vi "AlliGator Script Sequential ROIs Time-Gated Data Series Phasor Analysis.vi"(6 "AlliGator Data Series Type":T9, 8 "Error In":errorcluster, 9 "AlliGator Ctrl Refnums":T1, 10 "Path":path, 11 "Alligator Queue Elements in":T10[](array[typedef])) -> (0 "Error Out":errorcluster, 1 "Message":string, 2 "Time-Series Paths":path[](array[path]), 3 "Alligator Queue Elements out":T10[](array[typedef]))   [LabVIEW 2021, in "AlliGator Scripts.lvlib"]
doc: "Script performing phasor analysis of a different ROI for each dataset in a series. This is used for instance if the ROI list is representing the successive locations of an object being tracked across the dataset series."
uses:
  AlliGator Scripts.lvlib
  AlliGator Q Event.ctl
  AlliGator Action Engine.lvlib
  AlliGator Q Element.ctl
  Alligator Elements Order in Action Stack.ctl
  AlliGator Globals, Variables & Constants.lvlib
  AlliGator Variables List.ctl
  AlliGator Settings.lvlib
  AlliGator Settings List.ctl
  Graphs/XY Graph/XY Graph Plot Shift Method.ctl
  Graphs/XY Graph/XY Graph Add-Ons.lvlib
  Graphs/XY Graph/XY Graph Plot Shift Parameters.ctl
  Strings/Strings.lvlib
  Files/Files.lvlib
  AlliGator Phasor Ratio.lvlib
  AlliGator Files.lvlib
  AlliGator FLI Dataset Type.ctl
  AlliGator Add Action Array to Stack.vi
  Graphs/Plot Scales.ctl
  Graphs/LabVIEW Plot Interpolation.ctl
  Graphs/Graphs.lvlib
  Graphs/Plot Point Style.ctl
  Graphs/XY Graph/New Plot Information.ctl
  AlliGator Displayed Image.ctl
  AlliGator Source Image.lvlib
  Phasor/Phasor Standard Deviation Options.ctl
  Phasor/Phasor.lvlib
  Phasor/Phasor Ratio Type.ctl
  Variant/Variant to Data/Variant to Data.lvlib
  Variant/Variant to Data/Variant to Boolean.vi
  AlliGator Add Single Action to Stack.vi
  AlliGator ROIs.lvlib
  AlliGator ROI Manager Actions.ctl
  AlliGator ROI Selection Data.ctl
  <vilib>/Utility/miscctls.llb/LVPoint32TypeDef.ctl
  Graphs/XY Graph/XY Graph Refnum.ctl
  Graphs/XY Graph/XY Graph Mouse Click Event Data.ctl
  AlliGator Phasor Ratio at Mouse Location Data.ctl
  AlliGator Data Series Type.ctl
  AlliGator Dataset Ctrl Refnums.ctl
  AlliGator GUI.lvlib
  AlliGator Registered Events Ctrl Refnums.ctl
  Phasor/Phasor Calibration Type.ctl
  AlliGator Phasor Graph Ctrl Refnums.ctl
  AlliGator Phasor Plot Ctrl Refnums.ctl
  AlliGator State Indicator.ctl
  AlliGator Other Ctrl Refnums.ctl
  Histograms/Histogram Bin Position.ctl
  Histograms/Histogram Window.lvlib
  Histograms/Histogram Bin Option.ctl
  Histograms/Linear Histogram Options.ctl
  AlliGator Image Histogram Control Refnums.ctl
  AlliGator Decay Fit Map Control Refnums.ctl
  AlliGator Decay Fit Parameter Map.lvlib
  AlliGator Ctrl Refnums.ctl
  Fits/IRF(X)PSED/Decay Fit Parameters & Derived Quantities List.ctl
  Fits/Fits.lvlib
  AlliGator Main Window Tabs.ctl
panel:
  out "# Time Points":i32
  # "see the AlliGator License on the block diagram (Ctrl+E or Window:Show Block Diagram)"
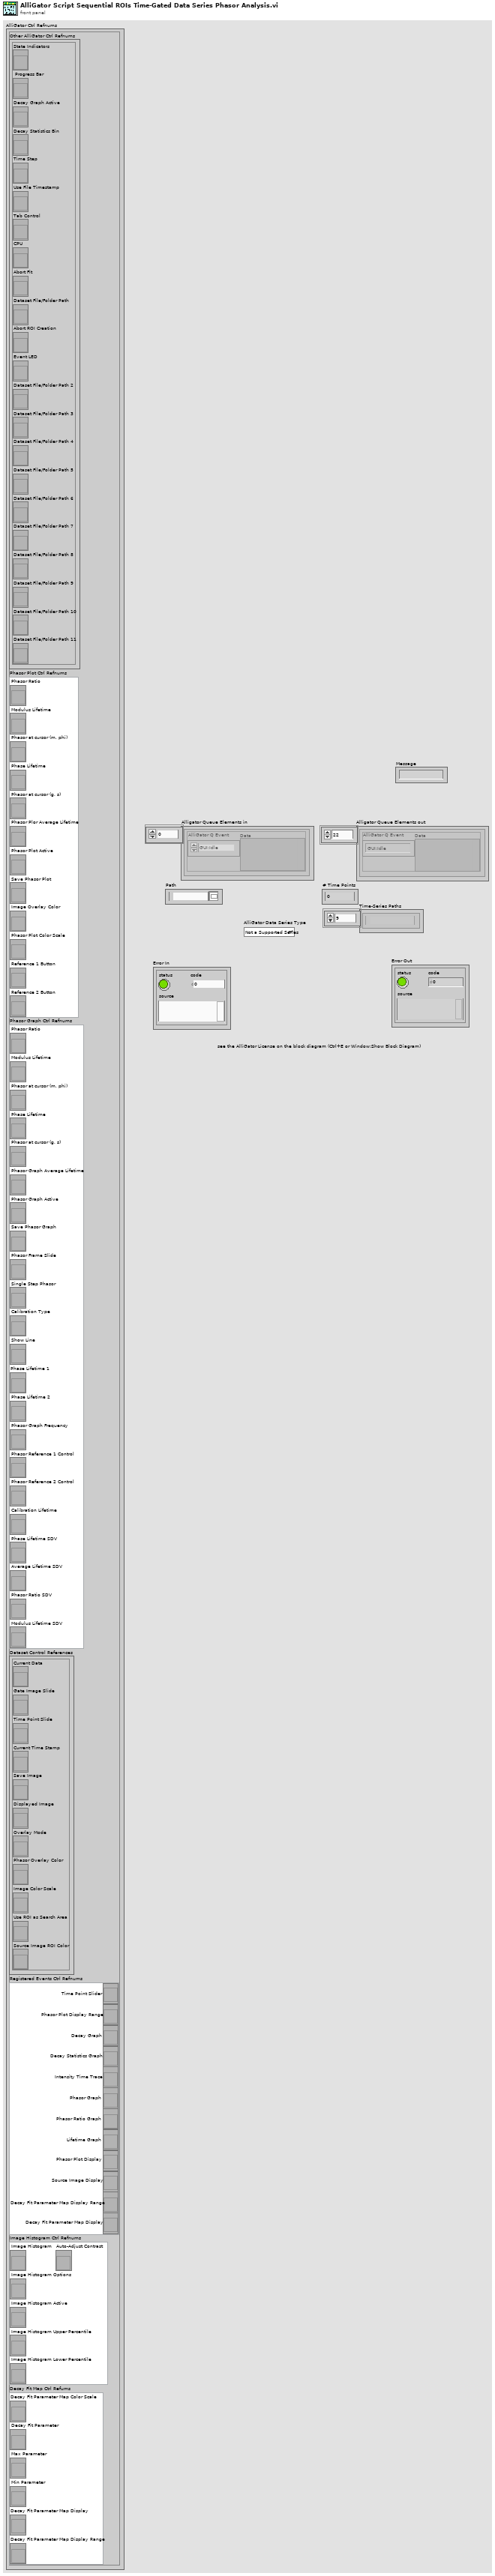
[diagram p1: front panel]
types:
  T1 = typedef "AlliGator GUI.lvlib/AlliGator Ctrl Refnums.ctl" = cluster{"Other AlliGator Ctrl Refnums":T2, "Phasor Plot Ctrl Refnums":T3, "Phasor Graph Ctrl Refnums":T4, "Dataset Control References":T5, "Registered Events Ctrl Refnums":T6, "Image Histogram Ctrl Refnums":T7, "Decay Fit Map Ctrl Refums":T8}
  T2 = typedef "AlliGator GUI.lvlib/AlliGator Other Ctrl Refnums.ctl" = cluster{"State Indicators":refnum<vi>, " Progress Bar":refnum<vi>, "Decay Graph Active":refnum<vi>, "Decay Statistics Bin":refnum<vi>, "Time Step":refnum<vi>, "Use File Timestamp":refnum<vi>, "Tab Control":refnum<vi>, "CPU":refnum<vi>, "Abort Fit":refnum<vi>, "Dataset File/Folder Path":refnum<vi>, "Abort ROI Creation":refnum<vi>, "Event LED":refnum<vi>, "Dataset File/Folder Path 2":refnum<vi>, "Dataset File/Folder Path 3":refnum<vi>, "Dataset File/Folder Path 4":refnum<vi>, "Dataset File/Folder Path 5":refnum<vi>, "Dataset File/Folder Path 6":refnum<vi>, "Dataset File/Folder Path 7":refnum<vi>, "Dataset File/Folder Path 8":refnum<vi>, "Dataset File/Folder Path 9":refnum<vi>, "Dataset File/Folder Path 10":refnum<vi>, "Dataset File/Folder Path 11":refnum<vi>}
  T3 = typedef "AlliGator GUI.lvlib/AlliGator Phasor Plot Ctrl Refnums.ctl" = cluster{"Phasor Ratio":refnum<vi>, "Modulus Lifetime":refnum<vi>, "Phasor at cursor (m, phi)":refnum<vi>, "Phase Lifetime":refnum<vi>, "Phasor at cursor (g, s)":refnum<vi>, "Phasor Plor Average Lifetime":refnum<vi>, "Phasor Plot Active":refnum<vi>, "Save Phasor Plot":refnum<vi>, "Image Overlay Color":refnum<vi>, "Phasor Plot Color Scale":refnum<vi>, "Reference 1 Button":refnum<vi>, "Reference 2 Button":refnum<vi>}
  T4 = typedef "AlliGator GUI.lvlib/AlliGator Phasor Graph Ctrl Refnums.ctl" = cluster{"Phasor Ratio":refnum<vi>, "Modulus Lifetime":refnum<vi>, "Phasor at cursor (m, phi)":refnum<vi>, "Phase Lifetime":refnum<vi>, "Phasor at cursor (g, s)":refnum<vi>, "Phasor Graph Average Lifetime":refnum<vi>, "Phasor Graph Active":refnum<vi>, "Save Phasor Graph":refnum<vi>, "Phasor Frame Slide":refnum<vi>, "Single Step Phasor":refnum<vi>, "Calibration Type":refnum<vi>, "Show Line":refnum<vi>, "Phase Lifetime 1":refnum<vi>, "Phase Lifetime 2":refnum<vi>, "Phasor Graph Frequency":refnum<vi>, "Phasor Reference 1 Control":refnum<vi>, "Phasor Reference 2 Control":refnum<vi>, "Calibration Lifetime":refnum<vi>, "Phase Lifetime SDV":refnum<vi>, "Average Lifetime SDV":refnum<vi>, "Phasor Ratio SDV":refnum<vi>, "Modulus Lifetime SDV":refnum<vi>}
  T5 = typedef "AlliGator GUI.lvlib/AlliGator Dataset Ctrl Refnums.ctl" = cluster{"Current Data":refnum<vi>, "Gate Image Slide":refnum<vi>, "Time Point Slide":refnum<vi>, "Current Time Stamp":refnum<vi>, "Save Image":refnum<vi>, "Displayed Image":refnum<vi>, "Overlay Mode":refnum<vi>, "Phasor Overlay Color":refnum<vi>, "Image Color Scale":refnum<vi>, "Use ROI as Search Area":refnum<vi>, "Source Image ROI Color":refnum<vi>}
  T6 = typedef "AlliGator GUI.lvlib/AlliGator Registered Events Ctrl Refnums.ctl" = cluster{"Time Point Slider":refnum<vi>, "Phasor Plot Display Range":refnum<vi>, "Decay Graph":refnum<vi>, "Decay Statistics Graph":refnum<vi>, "Intensity Time Trace":refnum<vi>, "Phasor Graph":refnum<vi>, "Phasor Ratio Graph":refnum<vi>, "Lifetime Graph":refnum<vi>, "Phasor Plot Display":refnum<vi>, "Source Image Display":refnum<vi>, "Decay Fit Parameter Map Display Range":refnum<vi>, "Decay Fit Parameter Map Display":refnum<vi>}
  T7 = typedef "AlliGator GUI.lvlib/AlliGator Image Histogram Control Refnums.ctl" = cluster{"Image Histogram":refnum<vi>, "Image Histogram Options":refnum<vi>, "Image Histogram Active":refnum<vi>, "Image Histogram Upper Percentile":refnum<vi>, "Image Histogram Lower Percentile":refnum<vi>, "Auto-Adjust Contrast":refnum<vi>}
  T8 = typedef "AlliGator Decay Fit Parameter Map.lvlib/AlliGator Decay Fit Map Control Refnums.ctl" = cluster{"Decay Fit Parameter Map Color Scale":refnum<vi>, "Decay Fit Parameter":refnum<vi>, "Max Parameter":refnum<vi>, "Min Parameter":refnum<vi>, "Decay Fit Parameter Map Display":refnum<vi>, "Decay Fit Parameter Map Display Range":refnum<vi>}
  T9 = typedef "AlliGator Files.lvlib/AlliGator Data Series Type.ctl" = enum16{"Not a Supported Series", "Gate Images Folder Series", "SwissSPAD 2 Dataset Series", "B&H FLI Dataset Series", "PicoQuant PTU FLI Dataset Series", "PicoQuant BIN FLI Dataset Series", "Piccolo hist BIN FLI Dataset Series", "HDF5 FLI Dataset Series"}
  T10 = typedef "AlliGator Action Engine.lvlib/AlliGator Q Element.ctl" = cluster{"AlliGator Q Event":T11, "Data":variant}
  T11 = typedef "AlliGator Action Engine.lvlib/AlliGator Q Event.ctl" = enum16{"---- Files ----", "Files:Set Batch Export Files To Save", "Files:Set Dataset Loading & Pre-processing Options", "Files:Check #Frames in Dataset", "Files:Increment Frame Index", "Files:Open Mask Image", "Files:Open White Light Image", "Files:Open Single Dataset", "Files:New Folder of Folders Selected", "Files:Load File (all Types)_Scriptable", "Files:Move Flattened Series to Folders Series", "Files:Select Folder", "Files:Load FLI Dataset", "Files:Load Swiss SPAD 1 Dataset", "Files:Load Swiss SPAD 2 Dataset", "Files:Load .sdt FLI Dataset", "Files:Load .ptu FLI Dataset", "Files:Load .bin FLI Dataset", "Files:Load Single Gate Image Folder", "Files:Load I/m/phi Dataset (deprecated)", "Files:Load Single Image", "Files:Subtract Background File", "Files:Export FLI Dataset", "Files:Load HDF5 FLI Dataset", "Files:Set Destination File Path", "Files:Save Mask Image", "Files:Batch Conversion", "Files:New Folder Selected", "Files:Close FLI Dataset", "Files:Close FLI Dataset Series", "Files:Close White Light Image", "Files:Close Mask Image", "---- FLI Dataset ----", "FLI Dataset:Channel Arithmetic", "FLI Dataset:Export Average Lifetime Map as ASCII", "FLI Dataset:Export User-Defined Quantity Map as ASCII", "FLI Dataset:Python Function FLI Dataset Event", "FLI Dataset:ROI Analysis", "FLI Dataset:Tilted Logistic Square Gated IRF Characteristics Map", "FLI Dataset:Logistic Square Gated IRF Characteristics Map", "FLI Dataset:Square Gated IRF Characteristics Map", "FLI Dataset:Multi-ROI Single-Pixel Phasor Analysis", "FLI Dataset:Multi-ROI Single-Pixel NLSF Analysis", "FLI Dataset:All ROIs IRF Extraction", "FLI Dataset:All ROIs Decay Fit Non-Interactive (Fast + Individual IRF)", "FLI Dataset:All ROIs Phasor Analysis", "FLI Dataset:All ROIs Decay Fit", "FLI Dataset:Fluorescence Decay Statistics", "FLI Dataset:Update Decay Statistics Graph", "FLI Dataset:Get Decay from ROI", "FLI Dataset:All ROIs Average Lifetimes", "---- FLI Dataset Series ----", "FLI Dataset Series:Sum All Datasets in Series", "FLI Dataset Series:Add Dataset to Accumulated Dataset", "FLI Dataset Series:Display Accumulated Dataset", "FLI Dataset Series:Clear Dataset Series Sum", "FLI Dataset Series:Time-Series Analysis (NLSF)", "FLI Dataset Series:Time-Series Analysis (Phasor)", "---- Image ----", "Image:Update Image Profile Plots", "Image:Image Histogram Cursor Move", "Image:Image Histogram", "Image:Image Contrast", "Image:Set Image Histogram Cursor Move Flag", "Image:Clear Image Overlay", "Image:Use ROI as Search Area", "Image:Set ROI Diameter", "Image:Save Image Data as TIFF", "Image:Save Displayed Image with Overlay", "Image:Save Image Overlay Only", "Image:Save Image as Hot Pixel Mask", "Image:Change Source Image Color Palette", "Image:Copy Image to Clipboard", "Image:Source Image ROI Selection", "Image:Delete All ROIs", "Image:Delete All Unselected ROIs", "Image:Delete ROI", "Image:Merge All ROIs", "Image:Store ROI", "Image:Source Image ROI Storage", "Image:Export ROI Description to Notebook", "Image:Save ROI", "Image:Load ROI", "Image:Paste ROI Definition", "Image:Clear ROI", "Image:Identify ROIs in Mask Image", "Image:Create Complementary ROI", "Image:Create Contour ROI", "Image:Create ROI(s) from Pixels with Peak above Min_Scriptable", "Image:Create ROI(s) from Pixels with Intensity above Min_Scriptable", "Image:Compute ROI Statistics", "Image:Delete ROI(s) based on ROI Characteristics", "Image:Create ROI Grid", "Image:ROI to Individual Pixel ROIs", "Image:Python Function Source Image Event", "Image:Show Phasor Calibration Map ROI Centers", "Image:Convert ROI to Mask Image", "Image:Mouse Move", "Image:Mouse Up", "Image:Set Source Image Mouse Move Flag", "Image:Add Scale Bar Overlay", "Image:Delete Existing ROIs Option", "---- Decay ----", "Decay:Clear IRF/Reference Plot", "Decay:Clear Local IRFs", "Decay:Add Decay to Graph", "Decay:Smoothen Plot", "Decay:Smoothen Plot Tail", "Decay:Average Selected Plots", "Decay:Extract IRF", "Decay:Optimal IRF Extraction", "Decay:Threshold IRF", "Decay:Fit to Model IRF", "Decay:Fit IRF to Square Gate", "Decay:Fit IRF to Logistic Square Gate", "Decay:Fit IRF to Tilted Logistic Square Gate", "Decay:Create Bounding Cursors Set", "Decay:Export Bounding Cursors Definition to Notebook", "Decay:Denoise Plot", "Decay:Compute Cumulative Function", "Decay:Use as Reference Decay", "Decay:Show Reference Decay/IRF", "Decay:Extrapolate Decay", "Decay:Create Head & Tail Bounding Cursors", "Decay:Store Cursor-defined Head & Tail Fractions", "Decay:Rebin Plot", "Decay:1-Normalize Decay", "Decay:[0-1]-Normalize Plot", "Decay:Straighten Decay", "Decay:Shift Decay", "Decay:Fold Decay", "Decay:Fit Decay", "Decay:Global Fit of Selected Decays", "Decay:Post Global Fit Script", "Decay:Add Global Fit Parameters to Graph", "Decay:Add Decay Parameter(s) to Plot (Graph)", "Decay:Export Decay to Phasor Graph", "Decay:Plot Decay Shifts", "Decay:Compute Average Lifetime", "Decay:Plot Convolution", "Decay:Graph Tip Strip Update", "---- Decay Statistics ----", "Decay Statistics:Tip Strip Update", "---- Intensity Time Trace ----", "Intensity Time Trace:Use File Timestamp", "Intensity Time Trace:Load Intensity Corrections File", "Intensity Time Trace:Clear Intensity Corrections File", "Intensity Time Trace:Tip Strip Update", "---- Phasor Plot ----", "Phasor Plot:Build Phasor Plot", "Phasor Plot:Change Phasor Plot Color Palette", "Phasor Plot:Adjust Phasor Plot Display Range", "Phasor Plot:Highlight Image ROI in Phasor Plot", "Phasor Plot:Save Phasor Plot Image with Overlay", "Phasor Plot:Export Complex Phasor Map", "Phasor Plot:Export Phasor Ratio Map", "Phasor Plot:Export Average Lifetime Map", "Phasor Plot:Compute Phase Lifetime Histogram", "Phasor Plot:Compute Phasor Ratio Histogram", "Phasor Plot:Compute Phase Lifetime vs Intensity Scatter Plot", "Phasor Plot:Weber 2-Component Decomposition", "Phasor Plot:Update Phasor Color Map Vertices", "Phasor Plot:Clear Phasor Overlay", "Phasor Plot:Use Segment Extremities as References", "Phasor Plot:Use UC/Segment Intersections as References", "Phasor Plot:Use UC/Principal Axis Intersections as References", "Phasor Plot:Use UC/Linear Fit Intersections as References", "Phasor Plot:Update Phasor Plot Reference", "Phasor Plot:Show Local Phasor Info in Phasor Plot", "Phasor Plot:Update Phasor Plot State", "Phasor Plot:Phasor Plot ROI Storage", "Phasor Plot:Phasor Plot ROI Selection", "Phasor Plot:Python Function Phasor Plot Event", "Phasor Plot:Overlay Phasor ROI, Ratio or Map in Source Image", "Phasor Plot:Compute Decay of Selected Phasors", "Phasor Plot:Phasor at Image Pixel", "Phasor Plot:Mouse Move", "Phasor Plot:Mouse Up", "Phasor Plot:Display Range Mouse Move", "Phasor Plot:Set Mouse Move Flag", "---- Phasor Graph ----", "Phasor Graph:Calibrated Phasor Map Series", "Phasor Graph:Whole Image Phasor Scatter Plot (Todo)", "Phasor Graph:Get Phasor Value", "Phasor Graph:Create New Phasor Plot Dialog", "Phasor Graph:Update Last Phasor Value", "Phasor Graph:Update Phasor (m, phi)", "Phasor Graph:Remove Single Phasor from Plot", "Phasor Graph:Add Single Phasor to Plot", "Phasor Graph:Remove Phasor Plot", "Phasor Graph:Remove Selected Phasor Plots", "Phasor Graph:Clear Phasor Data", "Phasor Graph:Clear Phasor Graph", "Phasor Graph:Cursor Move", "Phasor Graph:Draw Cursor Connecting Line", "Phasor Graph:Clear Cursor Connecting Line", "Phasor Graph:Find UC Intersection", "Phasor Graph:Use UC/Cursor-Defined Line Intersections", "Phasor Graph:Use Selected Plots Fitted Line/UC Intersections", "Phasor Graph:Use Selected Plots Principal Axis/UC Intersections", "Phasor Graph:Show Single Phasor", "Phasor Graph:Save Single Phasor Plot", "Phasor Graph:Save All Phasor Plots", "Phasor Graph:Load Phasor Plot(s)", "Phasor Graph:Phasor Multiplication", "Phasor Graph:Compute Average Phasor", "Phasor Graph:Compute Multiple Average Phasors (Selected Plots)", "Phasor Graph:Export Single Phasor Plot Phase Lifetimes", "Phasor Graph:Phase Lifetime Trajectory", "Phasor Graph:Phase Lifetime vs Intensity Scatter Plot (deprecated)", "Phasor Graph:Parameter 2 vs Parameter 1 Scatter Plot", "Phasor Graph:Use Cursor n Location", "Phasor Graph:Set Reference n to Current Phase Lifetime Value", "Phasor Graph:Set Reference n to Lifetime Value", "Phasor Graph:Set Cursor n Location", "Phasor Graph:Save Phasor Graph Image", "Phasor Graph:Update SEPL Plot", "Phasor Graph:Export Single Phasor Plot Data", "Phasor Graph:Export Selected Phasor Plots Data", "Phasor Graph:Python Function Phasor Graph Event", "Phasor Graph:Tip Strip Update", "---- Calibration ----", "Calibration:Set Calibration Type", "Calibration:Load/Save Phasor Calibration", "Calibration:Load/Save Phasor Calibration Series", "Calibration:Load/Save Phasor Calibration Map", "Calibration:Use as Calibration", "Calibration:Compute Optimal Calibration from Phasor References", "Calibration:Clear Phasor Calibration", "Calibration:Single Phasor Calibration Information", "Calibration:Use as Calibration Series", "Calibration:Use as Calibration Map", "Calibration:Clear Calibration Series", "Calibration:Phasor Calibration Series Information", "Calibration:Clear Calibration Map", "Calibration:Phasor Calibration Map Information", "Calibration:Apply Phasor Calibration", "Calibration:Update Single Plot Calibration", "Calibration:Update Multiple Plots Calibration", "Calibration:Clear Single Plot Calibration", "Calibration:Clear All Plots Calibrations", "Calibration:Clear Plot(s) Calibration(s)?", "Calibration:Phasor Calibration Maps (# Gates Series)", "---- Phasor Ratio ----", "Phasor Ratio:Clear Reference n", "Phasor Ratio:Toggle Selected Plot(s)  Lock to Reference 1", "Phasor Ratio:Use as Reference n", "Phasor Ratio:Send Reference n to Notebook", "Phasor Ratio:Toggle Selected Plot(s)  Lock to Reference 2", "Phasor Ratio:Compute Phasor Ratio at Mouse Location", "Phasor Ratio:Compute Phasor Plot's Average Phasor Ratio", "Phasor Ratio:Compute Time-Series Phasor Ratios", "Phasor Ratio:Fit Line to Phasor Ratio Plot", "Phasor Ratio:Save References", "Phasor Ratio:Load References", "Phasor Ratio:Update Phasor Reference 1", "Phasor Ratio:Update Phasor Reference 2", "Phasor Ratio:Move Cursor n to Reference n", "Phasor Ratio:Use as Phasor Reference 1 Lifetime", "Phasor Ratio:Use as Phasor Reference 2 Lifetime", "Phasor Ratio:Export Phasor Ratio Map as ASCII", "Phasor Ratio:Tip Strip Update", "---- Lifetime & Other Parameters Graph ----", "Lifetime:Tip Strip Update", "---- Decay Fit Parameter Map ----", "Decay Fit Parameter Map:Export ROI NLSF Data as ASCII", "Decay Fit Parameter Map:Set Decay Fit  Parameter Map Selection", "Decay Fit Parameter Map:Build Decay Fit Parameter Map", "Decay Fit Parameter Map:Change Decay Fit Parameter Map Color Palette", "Decay Fit Parameter Map:Export Decay Fit Parameter Map Data as ASCII", "Decay Fit Parameter Map:Export All Decay Fit Parameter Maps Data as ASCII", "Decay Fit Parameter Map:Send Map Data to Lifetime Graph", "Decay Fit Parameter Map:Save Decay Fit Parameter Map Image", "Decay Fit Parameter Map:Save-Load IRFs & Fit Data", "Decay Fit Parameter Map:Update Local Decay Plots", "Decay Fit Parameter Map:Python Function Decay Fit Parameters Map Event", "Decay Fit Parameter Map:Overlay Decay Fit Parameter Map in Source Image", "Decay Fit Parameter Map:Plot Map Data vs Intensity", "Decay Fit Parameter Map:Mouse Up", "Decay Fit Parameter Map:Display Range Mouse Move", "---- Generic Graph ----", "Generic Graph:Generic XY Graph Event", "Generic Graph:Python Function XY Graph Event", "Generic Graph:New Plot", "Generic Graph:Save Plot", "Generic Graph:XY Plot Histogram", "Generic Graph:Set XY Graph Plot Name", "Generic Graph:Set Last Cursor Style", "Generic Graph:Tip Strip Update", "---- GUI ----", "GUI:Start Script", "GUI:Type of Displayed Image Changed", "GUI:Gate Image Slide Changed", "GUI:Show Busy Icon", "GUI:Show Busy Icon & Abort Button", "GUI:Hide Busy Icon", "GUI:Hide Busy Icon & Abort Button", "GUI:Abort", "GUI:End Script", "GUI:Start Timing", "GUI:End Timing", "GUI:Set State Indicator", "GUI:Send Parameters JSON Strings to Clipboard", "GUI:Set Gate Step", "GUI:Idle", "GUI:Initialization", "GUI:Quit", "GUI:Increment Dataset Index", "GUI:Set Dataset Index to -1", "GUI:Time Series Slider Moved", "GUI:Time Series Slider Changed", "GUI:Toggle Playback or Loop", "GUI:Playback Script", "GUI:Set Phasor Frequency", "GUI:Open Window", "GUI:Start Test Script", "GUI:End Test Script", "DEBUG"}
  T12 = typedef "Phasor.lvlib/Phasor Ratio Type.ctl" = enum32{"Intensity-weighted", "Amplitude-weighted"}
  T13 = typedef "AlliGator Settings.lvlib/AlliGator Settings List.ctl" = enum16{"GUI:Visible Settings Tab", "GUI:Last Run Version", "Source Image:Use Image Histogram for Contrast", "Source Image:Low Count Pixels Rejection Options", "Source Image:High Count Pixels Rejection Options", "Source Image:Use Image Brightness", "Source Image:Blend Overlay with Image Background", "Source Image:Use Fixed ROI Diameter", "Source Image:ROI Diameter", "Source Image:ROI Center Color", "Source Image:Peak Threshold", "Source Image:Intensity Threshold", "Source Image:Image Binning Options", "Source Image:Image Smoothing Options", "Source Image:Image Histogram Active", "Source Image:Invert Binary Mask", "Source Image:Hot Pixel Removal", "Source Image:Overlay Analyzed ROI Center", "Source Image:Auto-Adjust Contrast", "Source Image:Histogram Lower Percentile", "Source Image:Histogram Upper Percentile", "Source Image:Save Source Image", "Source Image:Scale Bar Options", "Source Image:Image Resolution (Pixel Size)", "Source Image:Flatfield Correction", "Source Image:Show Dead Left Columns Correction", "Source Image:Dead Left Columns Correction", "Source Image:Image Pre-Processing Operations Order", "Data Information:Gate Width", "Data Information:Nanotime Gate Separation", "Data Information:Macrotime Gate Separation", "Data Information:Gate Step", "Data Information:# Gates", "Data Information:Gate Image Exposure", "Data Information:Gate Image Integration", "Data Information:Gates to Skip", "Data Information:Gates to Keep", "Data Information:Define Gates to", "Data Information:Channel Name", "Data Information:Available Channel Names", "Data Information:Channel Arithmetic", "Data Information:Background File Subtraction", "Data Information:Background File", "Data Information:Background Scaling Factor", "Data Information:Background Pile-up Correction", "Data Information:Background Pixel Well Capacity", "Data Information:Laser Period", "Data Information:SYNC Period", "Data Information:Pile-up Correction", "Data Information:Pixel Well Capacity", "Data Information:Dataset Scaling Factor", "Fluorescence Decay_Decay Pre-Processing:Reverse Gates", "Fluorescence Decay_Decay Pre-Processing:Verbose Decay Pre-Processing", "Fluorescence Decay_Decay Pre-Processing:Use Decay Pre-Processing", "Fluorescence Decay_Decay Pre-Processing:Background Subtraction", "Fluorescence Decay_Decay Pre-Processing:Background Definition Range", "Fluorescence Decay_Decay Pre-Processing:Baseline Subtraction Method", "Fluorescence Decay_Decay Pre-Processing:Decay Pre-Processing Operations Order", "Fluorescence Decay_Decay Pre-Processing:Smoothing Parameter", "Fluorescence Decay_Decay Pre-Processing:Shift Decay", "Fluorescence Decay_Decay Pre-Processing:Decay Shift Parameters", "Fluorescence Decay_Decay Pre-Processing:Fold Decay", "Fluorescence Decay_Decay Pre-Processing:# Folds", "Fluorescence Decay_Decay Pre-Processing:1-Normalize Decay", "Fluorescence Decay_Decay Pre-Processing:[0-1]-Normalize Decay", "Fluorescence Decay_Decay Pre-Processing:Smoothen Decay", "Fluorescence Decay_Decay Pre-Processing:Extrapolate Decay", "Fluorescence Decay_Decay Pre-Processing:Use Periodicity", "Fluorescence Decay_Decay Pre-Processing:Use Cursors", "Fluorescence Decay_Decay Pre-Processing:Tail Fraction", "Fluorescence Decay_Decay Pre-Processing:Head Fraction", "Fluorescence Decay_Decay Pre-Processing:Additional Points", "Fluorescence Decay_Decay Pre-Processing:Straighten Decay", "Fluorescence Decay_Decay Pre-Processing:Constant Background", "Fluorescence Decay_Decay Pre-Processing:Pixel-Normalize Decay", "Fluorescence Decay_Advanced Analysis:Extract IRF instead of Decay", "Fluorescence Decay_Advanced Analysis:IRF Extraction Options", "Fluorescence Decay_Advanced Analysis:IRF Optimization Options", "Fluorescence Decay_Advanced Analysis:Square Pulse Options", "Fluorescence Decay_Advanced Analysis:IRF Order", "Fluorescence Decay_Advanced Analysis:IRF Time Constants", "Fluorescence Decay_Advanced Analysis:Wavelet Analysis Options", "Fluorescence Decay_Advanced Analysis:Average Lifetime Options", "Fluorescence Decay_Fit Options:Fit Options", "Fluorescence Decay_Fit Options:Use Legacy Fitting Approach", "Fluorescence Decay_Fit Options:Use Data Information Laser Period", "Fluorescence Decay_Fit Parameters:Displayed Fit Parameters", "Fluorescence Decay_Fit Parameters:Fit Parameter Constraints", "Fluorescence Decay_Fit Parameters:Export Tabulated Results", "Fluorescence Decay_Fit Parameters:MLE Baseline Offset Type", "Fluorescence Decay_Fit Parameters:MLE Baseline Offset", "Fluorescence Decay_Fit Parameters:Guess Parameter Names", "Fluorescence Decay_Fit Parameters:Guess Parameter Values", "Fluorescence Decay_Fit Parameters:Guess Parameters Options", "Fluorescence Decay_Styles:Show Last Decay Only", "Fluorescence Decay_Styles:Decay Graph Color Array", "Fluorescence Decay:Decay Graph Active", "Fluorescence Decay Statistics:Min Peak Value", "Fluorescence Decay Statistics:Reject Low Decay Peak Pixels", "Fluorescence Decay Statistics:Reject High Decay Peak Pixels", "Fluorescence Decay Statistics:Max Peak Value", "Time Traces:Use File Timestamp", "Time Traces:Time Step", "Time Traces:Use Intensity Correction File", "Time Traces:Intensity Correction File", "Phasor Plot:Phasor Plot Smoothing Options", "Phasor Plot:Phasor Plot Size", "Phasor Plot:Phasor Plot Graphics Options", "Phasor Plot:Cumulative Phasor Plot", "Phasor Plot:Use Phasor Brightness", "Phasor Plot:Blend Overlay with Phasor Background", "Phasor Plot:Save Phasor Plot", "Phasor Plot:Show References", "Phasor Plot:Phasor Ratio Decay Range", "Phasor Plot:Exponential Fading", "Phasor Plot:Phasor Ratio Reference Colors", "Phasor Plot:Reference Radius", "Phasor Plot:Show Color Map Vertices", "Phasor Plot:Phasor Plot Active", "Phasor Plot:Phasor Ratio Color Map Type", "Phasor Plot:Phasor Ratio Color Map", "Phasor Plot:Phasor Ratio Display Range", "Phasor Plot:Selected Image ROI(s)", "Phasor Plot:All Image ROIs", "Phasor Plot:Selected Phasor Plot ROI(s)", "Phasor Plot:All Phasor Plot ROIs", "Phasor Plot:Phasor Ratio Color-Coded Quantity", "Phasor Plot:Store Phasor Harmonics", "Phasor Plot:Draw Reference Segment", "Phasor Plot:User-Defined Quantity", "Phasor Graph:Phasor Frequency", "Phasor Graph:Phasor Ratio Type", "Phasor Graph:Pixel-level Phasor Computation", "Phasor Graph:Save Phasor Graph", "Phasor Graph:Phasor Graph Active", "Phasor Graph:Phasor SDV Options", "Phasor Calibration:Use Backup Calibration if needed", "Phasor Graph:Define Shortest Lifetime as", "Phasor Calibration:Backup Calibration Type", "Phasor Calibration:Calibration Type", "Phasor Calibration:Calibration Lifetime", "Phasor Calibration:Calibration Map Algorithm", "Single-Exponential Phasor Locus (SEPL):Gate Parameters", "Single-Exponential Phasor Locus (SEPL):User-defined Gate", "Single-Exponential Phasor Locus (SEPL):User-defined IRF", "Single-Exponential Phasor Locus (SEPL):Phasor Parameters", "Single-Exponential Phasor Locus (SEPL):Decay & IRF Parameters", "Single-Exponential Phasor Locus (SEPL):Display Parameters", "Lifetime Analysis:Decay Analysis Parameters", "Lifetime Analysis:Lifetime Map Active", "Plugins:Python Settings", "Miscellaneous:Verbose Mode", "Miscellaneous:Beep after Script", "Miscellaneous:Saved Image File Format", "Miscellaneous:Exported Gate Image Settings", "Miscellaneous:Include Loading in Timing", "Miscellaneous:Verbose Settings Mode", "Miscellaneous:Histogram Options", "Miscellaneous:Beep on Error", "Miscellaneous:# Logical Processors Used", "Miscellaneous:ROI Description Max Characters", "Miscellaneous:Verbose Error Mode", "Miscellaneous:Transparent Mask Color"}
  T14 = typedef "Phasor.lvlib/Phasor Standard Deviation Options.ctl" = cluster{"Compute Estimated SDV":bool, "# Replicas":u32, "Use Estimated Average Phasor":bool}
  T15 = typedef "XY Graph Add-Ons.lvlib/XY Graph Plot Shift Method.ctl" = enum16{"Default", "CFD", "Threshold", "Cross-Correlation"}
  T16 = typedef "XY Graph Add-Ons.lvlib/XY Graph Plot Shift Parameters.ctl" = cluster{"Type":T15, "Shift":dbl[unit], "Threshold":dbl, "Rotate":bool}
  T17 = typedef "AlliGator Globals, Variables & Constants.lvlib/AlliGator Variables List.ctl" = enum16{"---- GUI ----", "GUI:Initialization Status", "GUI:State Indicators Refnum", "GUI:Original AlliGator Menu Items", "GUI:Current Action Loop State", "GUI:Script in progress", "GUI:Playback", "GUI:Loop Playback", "GUI:Search ROI Used", "GUI:Search ROI", "Decay Graph Max Legend Size", "Intensity Graph Max Legend Size", "Decay Statistics Graph Max Legend Size", "Phasor Graph Max Legend Size", "Phasor Ratio Graph Max Legend Size", "Lifetime Graph Max Legend Size", "---- Files ----", "Files:Export Dataset Frames as Individual Files", "Files:Show Batch Export Help Balloons", "Files:Frames in Dataset", "Files:ptu File Frame Start Indices", "Files:Current Frame in Dataset", "Files:Current Frame Timestamp", "Files:Dataset Loaded", "Files:Dataset Metadata", "Files:Dataset Channel", "Files:Dataset Data Description", "Files:Background Dataset Metadata", "Files:Background Dataset Channel", "Files:Background Dataset Data Description", "Files:Background File Subtraction", "Files:Background File Path", "Files:Background File Pile-up Correction", "Files:Background File Pixel Well Capacity", "Files:Background File Scaling Factor", "Files:Current Dataset Load Settings", "Files:Dataset Path", "Files:ICCD-specific Information", "Files:Macrotime Gate Separation", "------ Python Plugins ------", "Python Plugins:Information", "Python Plugins:Python Session", "Python Plugins:Valid Python Session?", "---- Source Image ----", "Source Image:ROIs", "Source Image:Current ROI", "Source Image:ROI Event Refnum", "X_Source Image Display Range", "X_Source Image Palette Information", "X_Type of Displayed Image", "X_Time Gate Slider", "Source Image:Palette List", "Source Image:Scale", "Source Image:ROI Overlay Color", "Source Image:Overlay to Erase", "Source Image:Is Displayed Image Accumulated", "Source Image:White Light Image Modified", "Source Image:Mask Image Modified", "---- Image Profile Window ----", "Image Profile:Overlay ROI in Source Image", "Image Profile:Window Event Refnum", "Image Profile:IntensityType", "Image Profile:Intensity Average Type", "Image Profile:Intensity-weighted SDV", "Image Profile:Box Profile Type", "Image Profile:Window Open", "Image Profile:Plotted Fit Parameter", "------ Phasor Graph -------", "Phasor Graph:Show Line", "---- Phasor Plot ---", "Phasor Plot:Parameters Changed", "Phasor Plot:FLI Dataset Modified since last Calculation", "Phasor Harmonics Data", "Selected Phasor Harmonics", "Phasor Harmonic Manager Event Refnum", "Phasor Plot:ROIs", "Phasor Plot:Current ROI", "Phasor Plot:ROI Event Refnum", "Phasor Plot:Image Reference Points", "Phasor Plot:Computed", "Phasor Plot:Palette Information", "Phasor Plot:Palette List", "Phasor Plot:Phasor Ratio Palette Information", "Phasor Plot:Phasor Ratio Palette List", "Phasor Plot:Image Scale", "Phasor Plot:Image Overlay to Erase", "Phasor Plot:Image Elements to Update", "Phasor Plot:Current Calculation Parameters", "Phasor Plot:Current Calibration Options", "Phasor Plot:Reset Cumulated Phasor Plot", "Phasor Plot:Reference 1", "Phasor Plot:Lifetime Reference 1", "Phasor Plot:Reference 1 Frequency", "Phasor Plot:Reference 2", "Phasor Plot:Lifetime Reference 2", "Phasor Plot:Reference 2 Frequency", "---- Decay Analysis ----", "Number of Selected Decays to Fit", "LS Fit Results", "LAR Fit Results", "BS Fit Results", "Last Decay Max - Min", "Best Fit Parameters", "Best Fit Parameter Names", "Actual Size X", "Actual Size Y", "Binning X", "Binning Y", "Actual # Gates", "Dataset Number", "Gates to...", "Gates Skipped", "Gates to keep", "Gate Step", "Gate Separation", "Reversed Gates", "Pile-up Correction", "Pixel Well Capacity", "Background Subtracted", "Background Subtraction Method", "Background Definition Range", "Background File (deprecated)", "Number of Dataset Accumulated", "Array of Accumulated Dataset Paths", "Do Averaged Datasets", "Destination File Path", "Process Plot Target", "Use 1/D as Phasor Frequency", "---- Decay Fit Parameter Map -----", "Decay Fit Parameter Map:Palette Information", "Decay Fit Parameter Map:Palette List", "------- Local Decay Window ---------", "Local Decay Graph Window:Event Refnum", "Local Decay Graph Window:Use normalized IRF for convolution", "----- Miscellaneous ----", "Misc:Skippable Dialog Windows Status"}
  T18 = enum16{"Start Script", "Load & Analyze Data", "End Script"}
  T19 = typedef "Phasor.lvlib/Phasor (g, s).ctl" = cluster{"g":dbl, "s":dbl}
  T20 = enum16{"None", "Reference 1", "Reference 2", "References 1 & 2"}
  T21 = typedef "AlliGator ROIs.lvlib/AlliGator ROI Selection Data.ctl" = cluster{"Action":T22, "ID":i32}
  T22 = typedef "AlliGator ROIs.lvlib/AlliGator ROI Manager Actions.ctl" = enum16{"Undefined", "Delete Current ROI", "Delete All Unselected ROIs", "Delete Multiple ROIs", "Delete All ROIs", "Swap ROIs", "Insert ROI", "Update Current ROI Descriptor", "Rename Current ROI", "Store New ROI", "Store Multiple ROIs", "Select Next ROI", "Select Previous ROI", "Find Selected ROI", "Show All ROIs", "Update ROI Manager Window", "Merge All ROIs", "Unmerge ROI", "Set Selected ROI by ID"}
  T23 = typedef "XY Graph Add-Ons.lvlib/New Plot Information.ctl" = cluster{"Multiplot XY Graph":refnum<vi>, "Plot Name":string, "Plot Scales":T24, "Plot Interpolation":T25, "Point Style":T26, "Plot Color":u32, "Plot Metadata":variant}
  T24 = typedef "XY Graph Add-Ons.lvlib/Plot Scales.ctl" = cluster{"X Scale":u32, "Y Scale":u32}
  T25 = typedef "Graphs.lvlib/LabVIEW Plot Interpolation.ctl" = u8
  T26 = typedef "Graphs.lvlib/Plot Point Style.ctl" = enum16{"not defined", "None", "Empty Circle", "Filled Circle", "Thick Circle", "Dotted Circle", "Empty Square", "Filled Square", "Thick Square", "Dotted Square", "Small Filled Square", "Dot", "Cross", "Tiny Cross", "Large X", "Small x", "Diamond", "Small Empty Square"}
  T27 = typedef "AlliGator Action Engine.lvlib/Alligator Elements Order in Action Stack.ctl" = enum16{"Enqueue 2 AFTER 1", "Enqueue 2 BEFORE 1"}
  T28 = typedef "AlliGator Source Image.lvlib/AlliGator Displayed Image.ctl" = enum16{"Single Gate", "Sum of All Gates", "Max of All Gates", "Min of All Gates", "-", "White Ligth Image", "Mask Image"}
  T29 = typedef "AlliGator Phasor Ratio.lvlib/AlliGator Phasor Ratio at Mouse Location Data.ctl" = cluster{"Mouse Click Event Data":T30, "Interactive?":bool}
  T30 = typedef "XY Graph Add-Ons.lvlib/XY Graph Mouse Click Event Data.ctl" = cluster{"Multiplot XY Graph":T31, "Mouse Coordinates":T32}
  T31 = typedef "XY Graph Add-Ons.lvlib/XY Graph Refnum.ctl" = refnum<vi>
  T32 = typedef "LVPoint32TypeDef.ctl" = cluster{"Horizontal":i32, "Vertical":i32}
  T33 = typedef "AlliGator Files.lvlib/AlliGator FLI Dataset Type.ctl" = enum16{"HDF5 FLI Dataset", "Gate Image Folder", ".sdt FLI Dataset (Becker & Hickl)", ".ptu FLI Dataset (PicoQuant)", "SS1 FLI Dataset", "SS2 FLI Dataset", "I/m/phi Dataset", ".bin FLI Dataset (PicoQuant Binned)", ".bin FLI Dataset (Piccolo Binned)"}
  T34 = typedef "AlliGator Displayed Image.ctl" = enum16{"Single Gate", "Sum of All Gates", "Max of All Gates", "Min of All Gates", "-", "White Ligth Image", "Mask Image"}
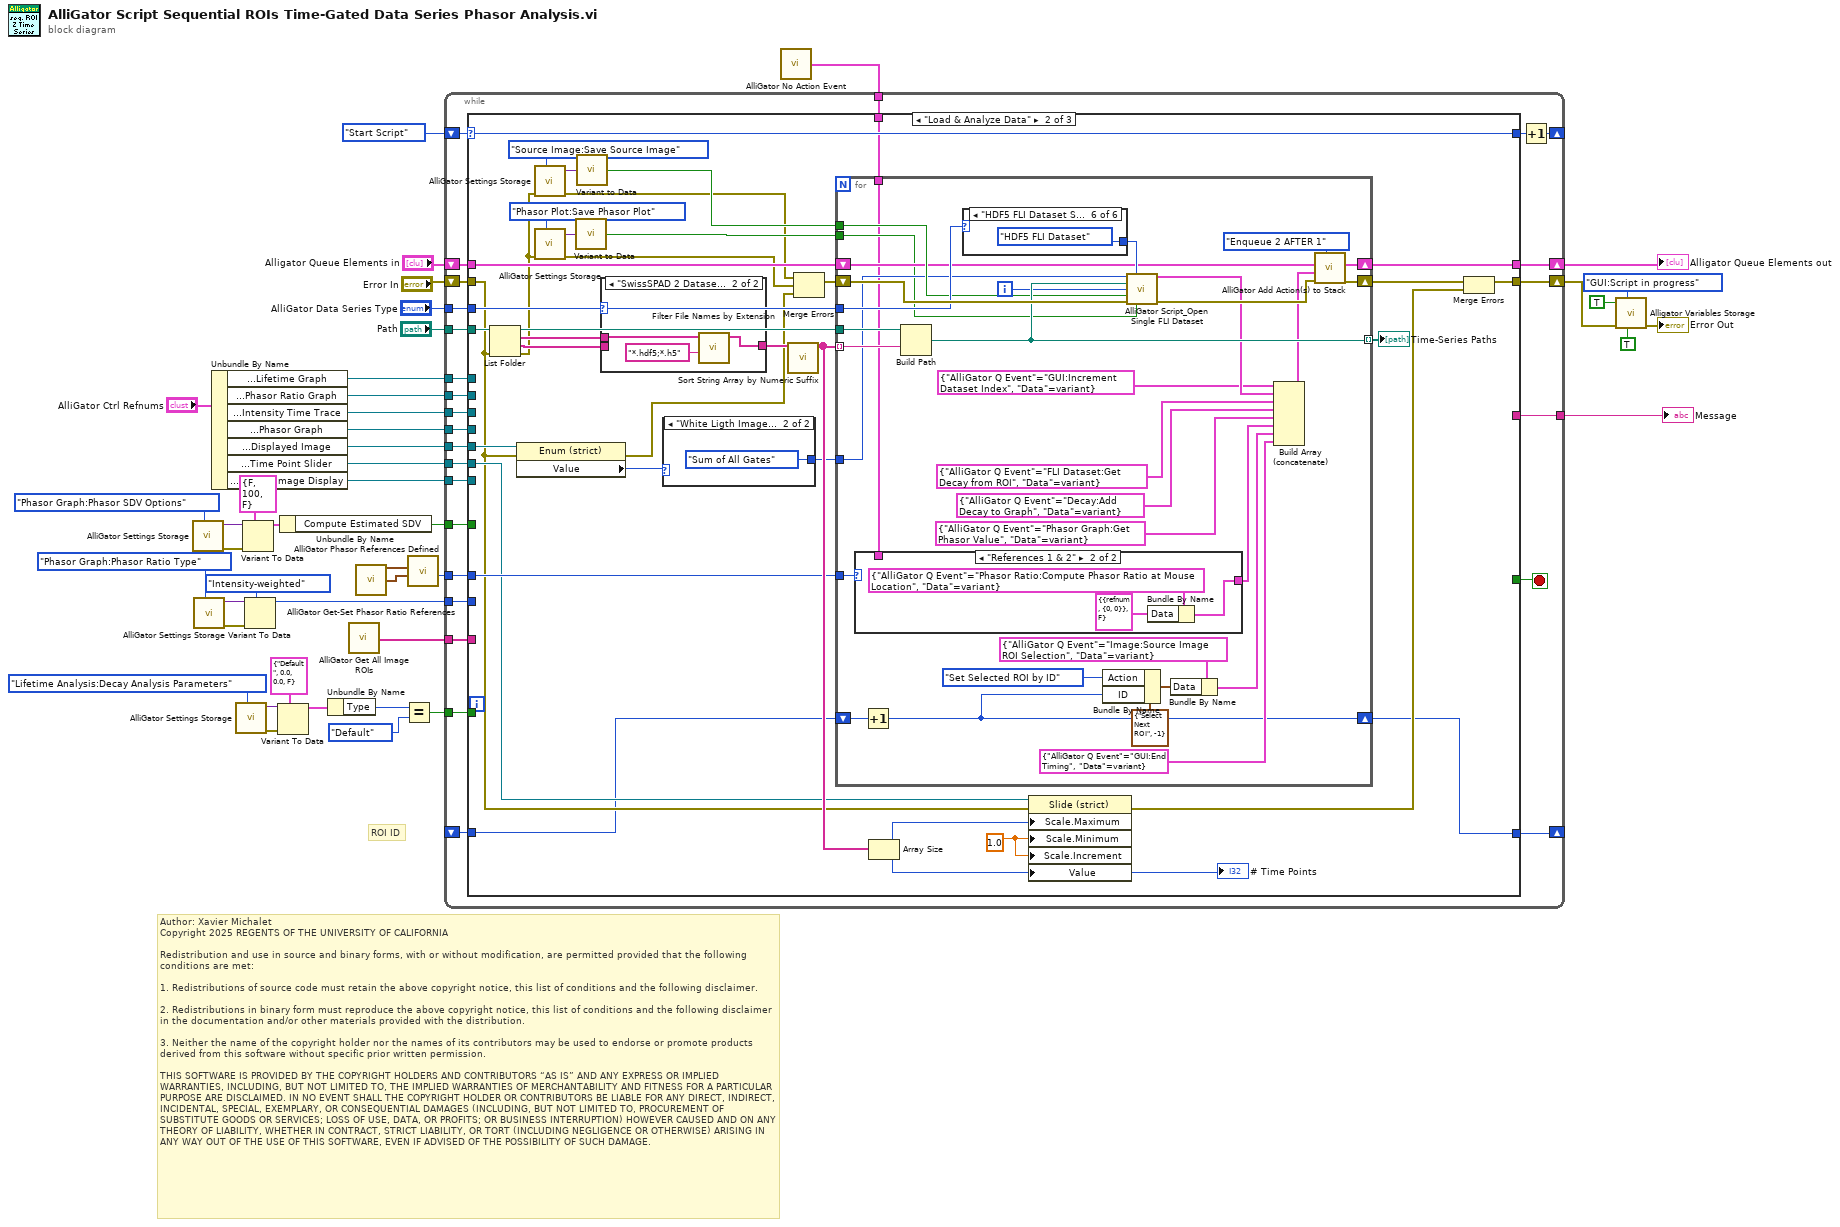
[diagram p0: block diagram]
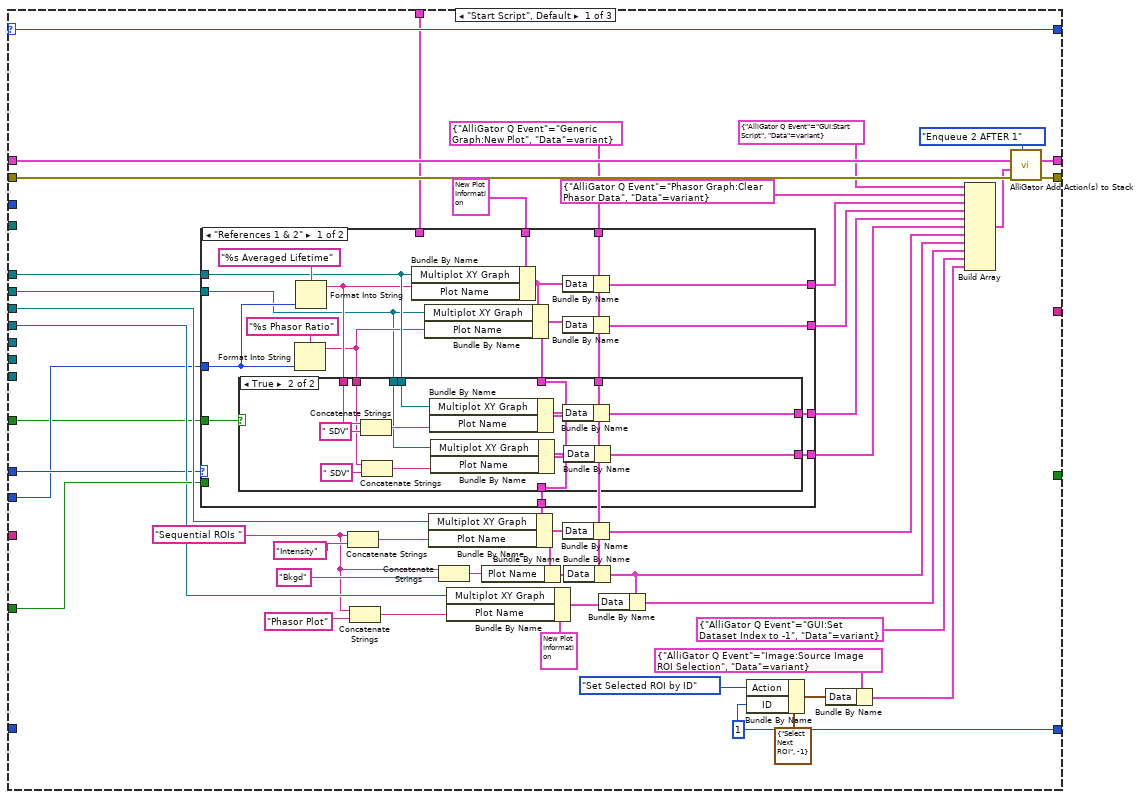
[diagram p2: hidden frame]
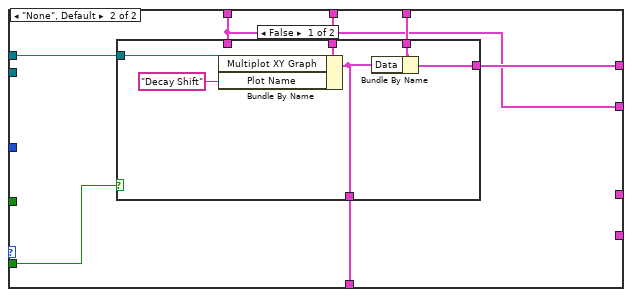
[diagram p4: hidden frame]
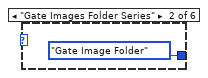
[diagram p10: hidden frame]
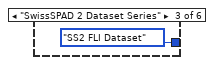
[diagram p11: hidden frame]
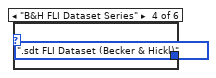
[diagram p12: hidden frame]
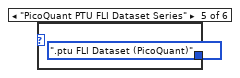
[diagram p13: hidden frame]
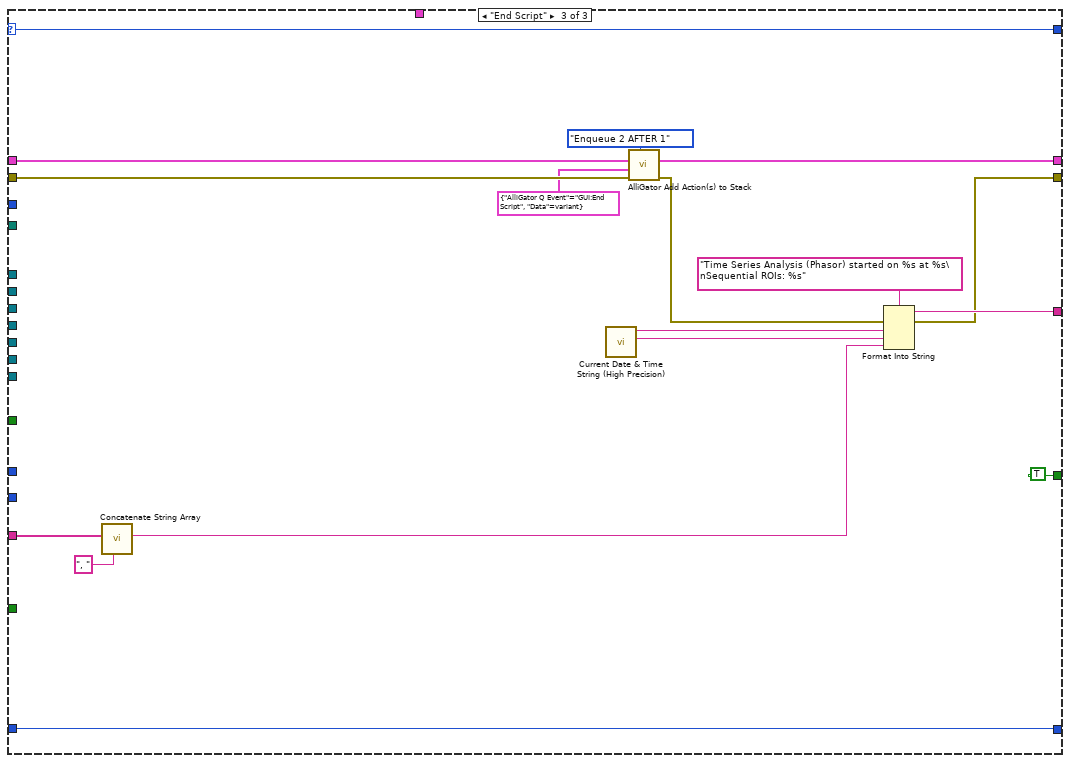
[diagram p14: hidden frame]
diagram:
  # "ROI ID"
  # "Author: Xavier Michalet\nCopyright 2025 REGENTS OF THE UNIVERSITY OF CALIFORNIA\n\nRedistribution and use in source and binary forms, with or without modification, are permitted provided that the following conditions are met:\n\n1. Redistributions of source code must retain the above copyright notice, this list of conditions and the following disclaimer.\n\n2. Redistributions in binary form must reproduce the above copyright notice, this list of conditions and the following disclaimer in the documentation and/or other materials provided with the distribution.\n\n3. Neither the name of the copyright holder nor the names of its contributors may be used to endorse or promote products derived from this software without specific prior written permission.\n\nTHIS SOFTWARE IS PROVIDED BY THE COPYRIGHT HOLDERS AND CONTRIBUTORS “AS IS” AND ANY EXPRESS OR IMPLIED WARRANTIES, INCLUDING, BUT NOT LIMITED TO, THE IMPLIED WARRANTIES OF MERCHANTABILITY AND FITNESS FOR A PARTICULAR PURPOSE ARE DISCLAIMED. IN NO EVENT SHALL THE COPYRIGHT HOLDER OR CONTRIBUTORS BE LIABLE FOR ANY DIRECT, INDIRECT, INCIDENTAL, SPECIAL, EXEMPLARY, OR CONSEQUENTIAL DAMAGES (INCLUDING, BUT NOT LIMITED TO, PROCUREMENT OF SUBSTITUTE GOODS OR SERVICES; LOSS OF USE, DATA, OR PROFITS; OR BUSINESS INTERRUPTION) HOWEVER CAUSED AND ON ANY THEORY OF LIABILITY, WHETHER IN CONTRACT, STRICT LIABILITY, OR TORT (INCLUDING NEGLIGENCE OR OTHERWISE) ARISING IN ANY WAY OUT OF THE USE OF THIS SOFTWARE, EVEN IF ADVISED OF THE POSSIBILITY OF SUCH DAMAGE."
  n1 = call "AlliGator Settings Storage.vi"("AlliGator Settings List"=AlliGator_Settings_List."Phasor Graph:Phasor SDV Options") -> ("Error Out"=w15:errorcluster, "Variant Data out"=w14:variant)  [unwired: 9 in]
  n2 = call "AlliGator Settings Storage.vi"("AlliGator Settings List"=AlliGator_Settings_List."Phasor Graph:Phasor Ratio Type") -> ("Error Out"=w8:errorcluster, "Variant Data out"=w9:variant)  [unwired: 9 in]
  n3 = Unbundle By Name("AlliGator Ctrl Refnums") -> ("Registered Events Ctrl Refnums.Lifetime Graph"=w32:refnum<vi>, "Registered Events Ctrl Refnums.Phasor Ratio Graph"=w33:refnum<vi>, "Registered Events Ctrl Refnums.Intensity Time Trace"=w34:refnum<vi>, "Registered Events Ctrl Refnums.Phasor Graph"=w23:refnum<vi>, "Dataset Control References.Displayed Image"=w3:refnum<vi>, "Registered Events Ctrl Refnums.Time Point Slider"=w4:refnum<vi>, "Registered Events Ctrl Refnums.Source Image Display"=w2:refnum<vi>)
  n4 = call "AlliGator Settings Storage.vi"("AlliGator Settings List"=AlliGator_Settings_List."Lifetime Analysis:Decay Analysis Parameters") -> ("Error Out"=w29:errorcluster, "Variant Data out"=w30:variant)  [unwired: 9 in]
  n5 = Variant To Data(error in=w15, type=T14 {"Compute Estimated SDV"=FALSE, "# Replicas"=100, "Use Estimated Average Phasor"=FALSE} ("Phasor SDV Options"), Variant=w14) -> (data=w12:T14)  [unwired: 1 out]
  n6 = Variant To Data(error in=w8, type=Phasor_Ratio_Type."Intensity-weighted" ("Phasor Ratio Type"), Variant=w9) -> (data=w6:T12)  [unwired: 1 out]
  n7 = Variant To Data(error in=w29, type=T16 {"Type"=enum."Default", "Shift"=0.0, "Threshold"=0.0, "Rotate"=FALSE} ("IRF Analysis Parameters"), Variant=w30) -> (data=w27:T16)  [unwired: 1 out]
  n8 = Unbundle By Name(w12) -> ("Compute Estimated SDV"=w11:bool)
  n9 = Unbundle By Name(w27) -> ("Type"=w25:T15)
  n10 = call "AlliGator Get All Image ROIs.vi"() -> ("ROI Names"=w1:string[])  [unwired: 9 in]
  n11 = call "AlliGator Get-Set Phasor Ratio References.vi"() -> ("Reference Phasor 1"=w19:T19, "Reference Phasor 2"=w20:T19)  [unwired: 8 in, 6 out]
  n12 = Equal?(x=w25, y=XY_Graph_Plot_Shift_Method."Default" ("Type")) -> (x = y?=w24:bool)
  n13 = call "AlliGator Phasor References Defined.vi"("Phasor Ratio Reference 2"=w20, "Phasor Ratio Reference 1"=w19) -> ("References Defined"=w18:T20)  [unwired: 9 in]
  n14 = call "AlliGator No Action Event.vi"() -> ("No Action"=w21:T10)
  n15 = while {
    tunnel: "Path" -> [w69]
    shift-right: [w66] -> w39
    shift-left: "Error In" -> [w70]
    shift-right: [w64] -> _
    shift-left: T18."Start Script" -> [w67]
    shift-right: [w62] -> w40
    shift-left: "Alligator Queue Elements in" -> [w68]
    tunnel: w34 -> [w61]
    tunnel: w33 -> [w60]
    tunnel: w32 -> [w59]
    tunnel: w24 -> [w58]
    tunnel: w23 -> [w57]
    tunnel: w1 -> [w56]
    tunnel: "AlliGator Data Series Type" -> [w55]
    tunnel: w21 -> [w54]
    tunnel: w18 -> [w53]
    tunnel: [w52] -> w17
    tunnel: w11 -> [w51]
    tunnel: w6 -> [w50]
    tunnel: w4 -> [w49]
    tunnel: w3 -> [w48]
    tunnel: w2 -> [w47]
    shift-right: [w46] -> _
    shift-left: _ -> [w45]
    stop <- w63 stop-if-true
    n16 = case shown="\"Load & Analyze Data\"" w67 {
      selector: w67 -> [w116 w198 w262]
      tunnel: w70 -> [w112 w177 w259]
      tunnel: w69 -> [_ w190 _]
      tunnel: w68 -> [w113 w199 w260]
      tunnel: [w114 w179 w251] -> w66
      tunnel: [w116 w198 w262] -> w65
      tunnel: [_ _ TRUE] -> w63
      tunnel: [w111 w196 w257] -> w62
      tunnel: w61 -> [w106 _ _]
      tunnel: w60 -> [w105 _ _]
      tunnel: w59 -> [w104 _ _]
      tunnel: w58 -> [w97 _ _]
      tunnel: w57 -> [w92 _ _]
      tunnel: w56 -> [_ _ w250]
      tunnel: w55 -> [_ w186 _]
      tunnel: w54 -> [w86 w184 _]
      tunnel: w53 -> [w85 w185 _]
      tunnel: [_ _ w253] -> w52
      tunnel: w51 -> [w80 _ _]
      tunnel: w50 -> [w81 _ _]
      tunnel: w49 -> [_ w182 _]
      tunnel: w48 -> [_ w181 _]
      tunnel: w47 -> [_ _ _]
      tunnel: [w71 w164 w247] -> w46
      tunnel: w45 -> [_ w165 w247]
      frame "Start Script", Default {
        w71 = 1
        w73 = "Sequential ROIs " ("t")
        w100 = T10 {"AlliGator Q Event"=enum."Generic Graph:New Plot", "Data"=variant} ("element")
        n17 = case shown="\"References 1 & 2\"" w85 {
          tunnel: [w133 w155] -> w108
          tunnel: [w132 w149] -> w107
          tunnel: w105 -> [w118 _]
          tunnel: w104 -> [w123 w154]
          tunnel: [w124 w151] -> w101
          tunnel: w100 -> [w121 w153]
          tunnel: T23 {"Multiplot XY Graph"=refnum, "Plot Name"="", "Plot Scales"={"X Scale"=0, "Y Scale"=0}, "Plot Interpolation"=7, "Point Style"=enum."not defined", "Plot Color"=15781887, "Plot Metadata"=variant} ("New Plot Information") -> [w130 w152]
          tunnel: w97 -> [_ w150]
          tunnel: w86 -> [_ w149]
          tunnel: w81 -> [w127 _]
          tunnel: w80 -> [w126 _]
          tunnel: [w120 _] -> w79
          tunnel: [w117 _] -> w78
          frame "References 1 & 2" {
            n18 = Format Into String(format string="%s Phasor Ratio" ("Plot Name"), w127) -> (resulting string=w119:string)  [unwired: 2 in, 1 out]
            n19 = Format Into String(format string="%s Averaged Lifetime" ("Plot Name"), w127) -> (resulting string=w122:string)  [unwired: 2 in, 1 out]
            n20 = Bundle By Name(cluster=w130, "Multiplot XY Graph"=w123, "Plot Name"=w122) -> (w131:T23)
            n21 = Bundle By Name(cluster=w131, "Multiplot XY Graph"=w118, "Plot Name"=w119) -> (w125:T23)
            n22 = case shown="True" w126 {
              tunnel: w125 -> [w134 w137]
              tunnel: [w134 w137] -> w124
              tunnel: w123 -> [_ w148]
              tunnel: w122 -> [_ w147]
              tunnel: w121 -> [_ w135]
              tunnel: [_ w143] -> w120
              tunnel: w119 -> [_ w139]
              tunnel: w118 -> [_ w138]
              tunnel: [_ w136] -> w117
              frame False {
              }
              frame True {
                n23 = Concatenate Strings(w147, " SDV" ("string")) -> (w146:string)
                n24 = Concatenate Strings(w139, " SDV" ("string")) -> (w140:string)
                n25 = Bundle By Name(cluster=w137, "Multiplot XY Graph"=w148, "Plot Name"=w146) -> (w144:T23)
                n26 = Bundle By Name(cluster=w137, "Multiplot XY Graph"=w138, "Plot Name"=w140) -> (w142:T23)
                n27 = Bundle By Name(cluster=w135, "Data"=w144) -> (w143:T10)
                n28 = Bundle By Name(cluster=w135, "Data"=w142) -> (w136:T10)
              }
            }
            n29 = Bundle By Name(cluster=w121, "Data"=w131) -> (w133:T10)
            n30 = Bundle By Name(cluster=w121, "Data"=w125) -> (w132:T10)
          }
          frame "None", Default {
            n31 = case shown="False" w150 {
              tunnel: [w161 w162] -> w155
              tunnel: w154 -> [w159 _]
              tunnel: w153 -> [w158 _]
              tunnel: w152 -> [w157 w163]
              tunnel: [w156 w163] -> w151
              tunnel: w149 -> [_ w162]
              frame False {
                n32 = Bundle By Name(cluster=w157, "Multiplot XY Graph"=w159, "Plot Name"="Decay Shift") -> (w156:T23)
                n33 = Bundle By Name(cluster=w158, "Data"=w156) -> (w161:T10)
              }
              frame True {
              }
            }
          }
        }
        n34 = Concatenate Strings(w73, "Intensity" ("Plot Name")) -> (w90:string)
        n35 = Concatenate Strings(w73, "Phasor Plot" ("Plot Name")) -> (w88:string)
        n36 = Bundle By Name(cluster=w101, "Multiplot XY Graph"=w106, "Plot Name"=w90) -> (w102:T23)
        n37 = Concatenate Strings(w73, "Bkgd" ("Plot Name")) -> (w89:string)
        n38 = Bundle By Name(cluster=T23 {"Multiplot XY Graph"=refnum, "Plot Name"="", "Plot Scales"={"X Scale"=0, "Y Scale"=0}, "Plot Interpolation"=0, "Point Style"=enum."Empty Circle", "Plot Color"=15781887, "Plot Metadata"=variant} ("New Plot Information"), "Multiplot XY Graph"=w92, "Plot Name"=w88) -> (w94:T23)
        n39 = Bundle By Name(cluster=w102, "Plot Name"=w89) -> (w95:T23)
        n40 = Bundle By Name(cluster=w100, "Data"=w102) -> (w99:T10)
        n41 = Bundle By Name(cluster=w100, "Data"=w95) -> (w96:T10)
        n42 = Bundle By Name(cluster=w96, "Data"=w94) -> (w93:T10)
        n43 = Bundle By Name(cluster=T21 {"Action"=enum."Select Next ROI", "ID"=-1} ("ROI Selection Data"), "Action"=AlliGator_ROI_Manager_Actions."Set Selected ROI by ID", "ID"=w71) -> (w77:T21)
        n44 = Bundle By Name(cluster=T10 {"AlliGator Q Event"=enum."Image:Source Image ROI Selection", "Data"=variant} ("Time-Gated Phasor Q Element"), "Data"=w77) -> (w74:T10)
        n45 = Build Array(T10 {"AlliGator Q Event"=enum."GUI:Start Script", "Data"=variant} ("element"), T10 {"AlliGator Q Event"=enum."Phasor Graph:Clear Phasor Data", "Data"=variant} ("element"), w108, w107, w79, w78, w99, w96, w93, T10 {"AlliGator Q Event"=enum."GUI:Set Dataset Index to -1", "Data"=variant} ("element"), w74) -> (w109:T10[])
        n46 = call-poly "AlliGator Add Action(s) to Stack.vi"("Elements Order in Action Stack (Default: 2 BEFORE 1)"=Alligator_Elements_Order_in_Action_Stack."Enqueue 2 AFTER 1", "Error In"=w112, "Alligator Queue Element 2"=w109, "Alligator Queue Element 1"=w113) -> ("Error Out"=w114:errorcluster, "Alligator Queue Element 1 (+ 2)"=w111:T10[])  [unwired: 6 in]
      }
      frame "Load & Analyze Data" {
        w195 = 1.0 ("Scale.Range:Minimum")
        n47 = List Folder(path=w190, error in=w177) -> (path out=w192:path, filenames=w189:string[], folder names=w188:string[], error out=w171:errorcluster)  [unwired: 2 in]
        n48 = property class="Enum (strict)"(reference=w181, error in=w177) -> (error out=w175:errorcluster, "Value"=w180:T34)  [unwired: 1 out]
        n49 = call "AlliGator Settings Storage.vi"("AlliGator Settings List"=AlliGator_Settings_List."Source Image:Save Source Image", "Error In"=w171) -> ("Error Out"=w168:errorcluster, "Variant Data out"=w170:variant)  [unwired: 8 in]
        n50 = call "AlliGator Settings Storage.vi"("AlliGator Settings List"=AlliGator_Settings_List."Phasor Plot:Save Phasor Plot", "Error In"=w171) -> ("Error Out"=w167:errorcluster, "Variant Data out"=w173:variant)  [unwired: 8 in]
        n51 = call-poly "Variant to Data.vi"("Variant"=w173) -> ("Value"=w172:bool)  [unwired: 8 in]
        n52 = call-poly "Variant to Data.vi"("Variant"=w170) -> ("Value"=w169:bool)  [unwired: 8 in]
        n53 = case shown="\"SwissSPAD 2 Dataset Series\", Default" w186 {
          tunnel: [w202 w203] -> w187
          tunnel: w189 -> [_ w205]
          tunnel: w188 -> [w202 _]
          frame "Gate Images Folder Series" {
          }
          frame "SwissSPAD 2 Dataset Series", Default {
            n54 = call "Filter File Names by Extension.vi"("patterns"="*.hdf5;*.h5", "filenames in"=w205) -> ("filenames out"=w203:string[])  [unwired: 7 in, 2 out]
          }
        }
        n55 = case shown="\"White Ligth Image\", \"Mask Image\"" w180 {
          selector: w180 -> [w200 _]
          tunnel: [w200 AlliGator_Displayed_Image."Sum of All Gates" ("Type of Displayed Image")] -> w183
          frame "Single Gate", Default {
          }
          frame "White Ligth Image", "Mask Image" {
          }
        }
        n56 = call "Sort String Array by Numeric Suffix.vi"("String Array"=w187) -> ("Sorted String Array"=w191:string[])  [unwired: 8 in, 2 out]
        n57 = Merge Errors(w168, w167, w175) -> (w176:errorcluster)
        n58 = for {
          shift-right: [w236] -> w196
          shift-left: w199 -> [w219]
          shift-right: [w232] -> w197
          shift-left: w176 -> [w231]
          tunnel: [w227] -> w193 mode=indexing
          tunnel: w191 -> [w228] mode=indexing
          tunnel: w192 -> [w229]
          tunnel: w186 -> [w225]
          tunnel: w169 -> [w222]
          tunnel: w172 -> [w215]
          tunnel: w185 -> [w214]
          tunnel: w184 -> [w213]
          tunnel: w183 -> [w217]
          shift-right: [w206] -> w164
          shift-left: w165 -> [w207]
          i -> [w216]
          n59 = case shown="\"References 1 & 2\"" w214 {
            tunnel: [w238 w240] -> w233
            tunnel: w213 -> [w238 _]
            frame "None", Default {
            }
            frame "References 1 & 2" {
              n60 = Bundle By Name(cluster=T10 {"AlliGator Q Event"=enum."Phasor Ratio:Compute Phasor Ratio at Mouse Location", "Data"=variant} ("element"), "Data"=T29 {"Mouse Click Event Data"={"Multiplot XY Graph"=refnum, "Mouse Coordinates"={"Horizontal"=0, "Vertical"=0}}, "Interactive?"=FALSE} ("output cluster")) -> (w240:T10)
            }
          }
          n61 = Increment(x=w207) -> (x+1=w206:i32)
          n62 = Build Path(base path=w229, name or relative path=w228) -> (appended path=w227:path)
          n63 = case shown="\"HDF5 FLI Dataset Series\"" w225 {
            tunnel: [_ AlliGator_FLI_Dataset_Type."Gate Image Folder" ("FLI Dataset Type") AlliGator_FLI_Dataset_Type."SS2 FLI Dataset" ("FLI Dataset Type") AlliGator_FLI_Dataset_Type.".sdt FLI Dataset (Becker & Hickl)" ("FLI Dataset Type") AlliGator_FLI_Dataset_Type.".ptu FLI Dataset (PicoQuant)" ("FLI Dataset Type") AlliGator_FLI_Dataset_Type."HDF5 FLI Dataset" ("FLI Dataset Type")] -> w224
            frame "Not a Supported Series", Default {
            }
            frame "Gate Images Folder Series" {
            }
            frame "SwissSPAD 2 Dataset Series" {
            }
            frame "B&H FLI Dataset Series" {
            }
            frame "PicoQuant PTU FLI Dataset Series" {
            }
            frame "HDF5 FLI Dataset Series" {
            }
          }
          n64 = Bundle By Name(cluster=T21 {"Action"=enum."Select Next ROI", "ID"=-1} ("ROI Selection Data"), "Action"=AlliGator_ROI_Manager_Actions."Set Selected ROI by ID", "ID"=w206) -> (w210:T21)
          n65 = call "AlliGator Script_Open Single FLI Dataset.vi"("Type of Displayed Image"=w217, "FLI Dataset Type"=w224, "File Path"=w227, "Dataset index in Series (0)"=w216, "Save Image with Overlay"=w222, "Error In"=w231, "Save Phasor Plot with Overlay"=w215) -> ("Action List out"=w221:T10[], "Error Out"=w226:errorcluster)  [unwired: 7 in]
          n66 = Bundle By Name(cluster=T10 {"AlliGator Q Event"=enum."Image:Source Image ROI Selection", "Data"=variant} ("Time-Gated Phasor Q Element"), "Data"=w210) -> (w209:T10)
          n67 = Build Array (concatenate)(T10 {"AlliGator Q Event"=enum."GUI:Increment Dataset Index", "Data"=variant} ("element"), w221, T10 {"AlliGator Q Event"=enum."FLI Dataset:Get Decay from ROI", "Data"=variant} ("element"), T10 {"AlliGator Q Event"=enum."Decay:Add Decay to Graph", "Data"=variant} ("element"), T10 {"AlliGator Q Event"=enum."Phasor Graph:Get Phasor Value", "Data"=variant} ("element"), w233, w209, T10 {"AlliGator Q Event"=enum."GUI:End Timing", "Data"=variant} ("element")) -> (w220:T10[])
          n68 = call-poly "AlliGator Add Action(s) to Stack.vi"("Elements Order in Action Stack (Default: 2 BEFORE 1)"=Alligator_Elements_Order_in_Action_Stack."Enqueue 2 AFTER 1", "Error In"=w226, "Alligator Queue Element 2"=w220, "Alligator Queue Element 1"=w219) -> ("Error Out"=w232:errorcluster, "Alligator Queue Element 1 (+ 2)"=w236:T10[])  [unwired: 6 in]
        }
        "Time-Series Paths" <- w193
        n69 = Array Size(array=w191) -> (size(s)=w194:i32)
        "# Time Points" <- w194
        n70 = property class="Slide (strict)"(reference=w182, error in=w177, "Scale.Maximum"=w194, "Scale.Minimum"=w195, "Scale.Increment"=w195, "Value"=w194) -> (error out=w178:errorcluster)  [unwired: 1 out]
        n71 = Merge Errors(w197, w178) -> (w179:errorcluster)
      }
      frame "End Script" {
        n72 = call "Concatenate String Array.vi"("Separator (TAB)"=", ", "String Array"=w250) -> ("Formatted String"=w248:string)  [unwired: 9 in]
        n73 = call "Current Date & Time String (High Precision).vi"() -> ("time string"=w254:string, "date string"=w255:string)  [unwired: 8 in, 2 out]
        n74 = call-poly "AlliGator Add Action(s) to Stack.vi"("Elements Order in Action Stack (Default: 2 BEFORE 1)"=Alligator_Elements_Order_in_Action_Stack."Enqueue 2 AFTER 1", "Error In"=w259, "Alligator Atomic Action"=T10 {"AlliGator Q Event"=enum."GUI:End Script", "Data"=variant} ("element"), "Alligator Queue Element 1"=w260) -> ("Error Out"=w252:errorcluster, "Alligator Queue Element 1 (+ 2)"=w257:T10[])  [unwired: 6 in]
        n75 = Format Into String(format string="Time Series Analysis (Phasor) started on %s at %s\nSequential ROIs: %s" ("initial string"), error in=w252, w255, w254, w248) -> (resulting string=w253:string, error out=w251:errorcluster)  [unwired: 1 in]
      }
    }
    n76 = Increment(x=w65) -> (x+1=w64:T18)
  }
  "Alligator Queue Elements out" <- w40
  "Message" <- w17
  n77 = call "Alligator Variables Storage.vi"("Get(F)/Set"=TRUE, "AlliGator Variable"=AlliGator_Variables_List."GUI:Script in progress" ("Alligator Variable"), "Error In"=w39, "Data in"=TRUE) -> ("Error Out"=→"Error Out":errorcluster)  [unwired: 5 in, 2 out]
